vi "Set Up Dialog - pH.vi"() -> ()   [LabVIEW 2012]
panel:
  out "Calibration Instructions":string="1. Connect the sensor to your myDAQ as shown in the diagram above.\n\n2. Take the boot off of the pH electrode and immerse in a 7.00pH buffer for 30 minutes.\n\n3. After 30 minutes is complete record the voltage to SP1\n\n4. Rinse off the electrode and immerse it in a 10.0pH buffer. The 30 minute wait does not need to be repeated here. Record the voltage for SP2."
  # "iWorx - pH - Set Up"
  # "pH Sensor (PHN - 100)"
  # "iWorx"
  # "Sensor"
  # "PHN - 100"
  # "myDAQ"
  # "Computer"
  # "Adaptor"
  # "Connection Diagram"
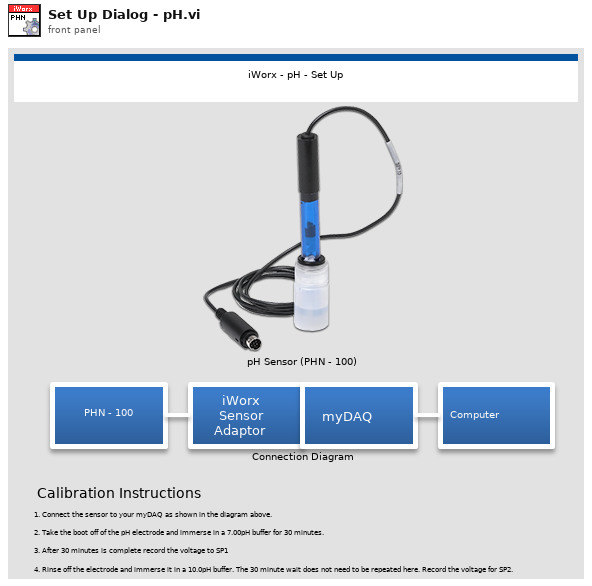
[diagram p1: front panel]
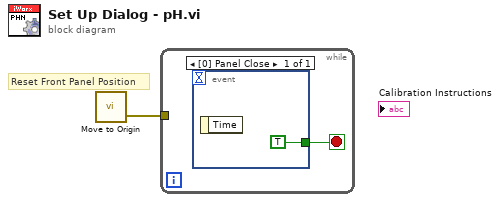
[diagram p0: block diagram]
diagram:
  # "Reset Front Panel Position"
  n1 = call "Move to Origin.vi"() -> ("Error Out"=w1:errorcluster)  [unwired: 3 in]
  n2 = while {
    tunnel: w1 -> [_]
    stop <- w2 stop-if-true
    n3 = event shown="[0] Panel Close" {
      selector: _ -> [_]
      dyn-events: _ -> [_]
      timeout: _ -> [_]
      tunnel: [TRUE] -> w2
      event Panel Close {
        n4 = event-data() -> ()  [unwired: 1 in, 1 out]
      }
    }
  }
